vi "save_chart_data.vi"(8 "error in (no error)":errorcluster, 11 "History Data":T1(array[cluster])) -> (0 "error out":errorcluster)   [LabVIEW 2018]
uses:
  <vilib>/Utility/file.llb/Write Delimited Spreadsheet (DBL).vi
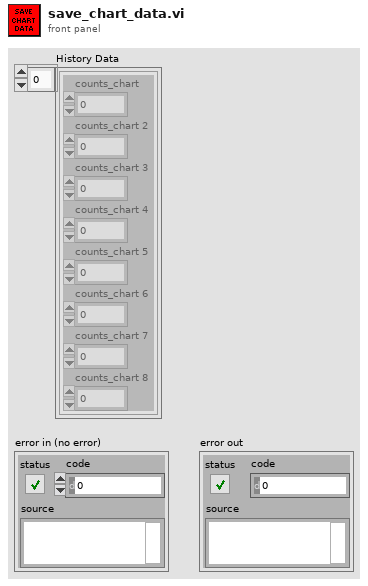
[diagram p1: front panel]
types:
  T1 = cluster{"counts_chart":dbl, "counts_chart 2":dbl, "counts_chart 3":dbl, "counts_chart 4":dbl, "counts_chart 5":dbl, "counts_chart 6":dbl, "counts_chart 7":dbl, "counts_chart 8":dbl}[]
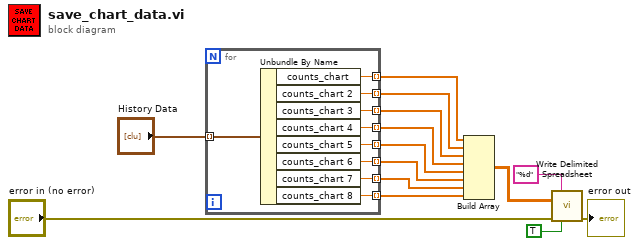
[diagram p0: block diagram]
diagram:
  n1 = for {
    tunnel: "History Data" -> [w23] mode=indexing
    tunnel: [w22] -> w3 mode=indexing
    tunnel: [w21] -> w6 mode=indexing
    tunnel: [w20] -> w5 mode=indexing
    tunnel: [w19] -> w4 mode=indexing
    tunnel: [w18] -> w10 mode=indexing
    tunnel: [w17] -> w9 mode=indexing
    tunnel: [w16] -> w7 mode=indexing
    tunnel: [w15] -> w8 mode=indexing
    n2 = Unbundle By Name(w23) -> ("counts_chart"=w22:dbl, "counts_chart 2"=w19:dbl, "counts_chart 3"=w20:dbl, "counts_chart 4"=w21:dbl, "counts_chart 5"=w16:dbl, "counts_chart 6"=w17:dbl, "counts_chart 7"=w18:dbl, "counts_chart 8"=w15:dbl)
  }
  n3 = Build Array(w3, w4, w5, w6, w7, w9, w10, w8) -> (w11:dbl[][])
  n4 = call-poly <vilib>:"Write Delimited Spreadsheet.vi"("format (%.3f)"="%d", "2D data"=w11, "error in (no error)"="error in (no error)", "transpose? (no:F)"=TRUE ("transpose? (F)")) -> ("error out"=→"error out":errorcluster)  [unwired: 10 in, 1 out]
